vi "Teardown Created Events.vi"(11 "qqqqq in":refnum<class "qqqqq.lvclass">) -> (3 "qqqqq out":refnum<class "qqqqq.lvclass">)   [LabVIEW 2021, in "Providers.lvlib" / "qqqqq.lvlib" / "qqqqq.lvclass"]
uses:
  qqqqq.lvclass
  qqqqq.lvclass/qqqqq.ctl
  jettl/Queue/Queue.lvclass
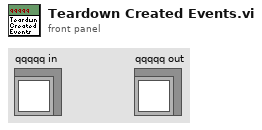
[diagram p1: front panel]
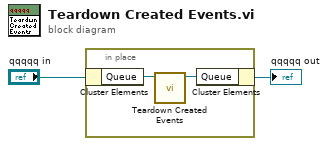
[diagram p0: block diagram]
diagram:
  n1 = in-place {
    n2 = in-place-cluster #1("qqqqq in") -> ("Queue"=w4:refnum<class "Queue.lvclass">)
    n3 = call-dynamic "Teardown Created Events.vi"("Queue in"=w4) -> ("Queue out"=w3:refnum<class "Queue.lvclass">)  [unwired: 10 in]
    n4 = in-place-cluster #1("Queue"=w3) -> (→"qqqqq out":refnum<class "qqqqq.lvclass">)
  }
